vi "Set Echo On.vi"(8 "error in (no error)":errorcluster, 11 "VISA resource name":refnum<visa-resource-name>="COM1") -> (0 "error out":errorcluster, 2 "query output":string, 3 "VISA resource name out":refnum<visa-resource-name>)   [LabVIEW 2017]
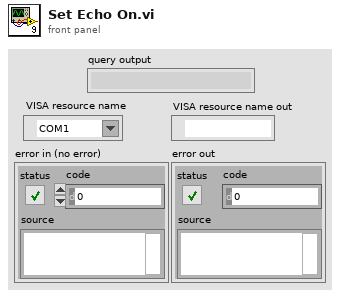
[diagram p1: front panel]
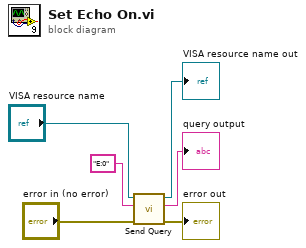
[diagram p0: block diagram]
diagram:
  n1 = call "Send Query.vi"("error in (no error)"="error in (no error)", "query string"="E:0", "VISA resource name"="VISA resource name") -> ("error out"=→"error out":errorcluster, "query output"=→"query output":string, "VISA resource name out"=→"VISA resource name out":refnum<visa-resource-name>)  [unwired: 6 in]
